vi "串口发送.vi"(6 "写入缓冲区":string, 7 "命令":string(combo), 8 "error in (no error)":errorcluster caption="错误输入（无错误）", 10 "baud rate (9600)":u32=115200 caption="波特率(115200)", 11 "VISA resource name":refnum<visa-resource-name> caption="VISA资源名称") -> (0 "错误输出":errorcluster, 3 "VISA resource name 2":refnum<visa-resource-name>, 4 "读取缓冲区":string)   [LabVIEW 2016]
uses:
  <vilib>/Instr/_visa.llb/VISA Flush IO Buffer Mask.ctl
  <vilib>/Instr/_visa.llb/VISA Configure Serial Port (Instr).vi
panel:
  in  "timeout (10sec)":u32=10000 caption="超时（10秒）"
  out "返回数":u32
  in  "parity (0:none)":enum16{"None", "Odd", "Even", "Mark", "Space"}(ring) caption="奇偶（0:无）"
  in  "data bits (8)":u16=8 caption="数据比特(8)" min=5 max=8 step=1
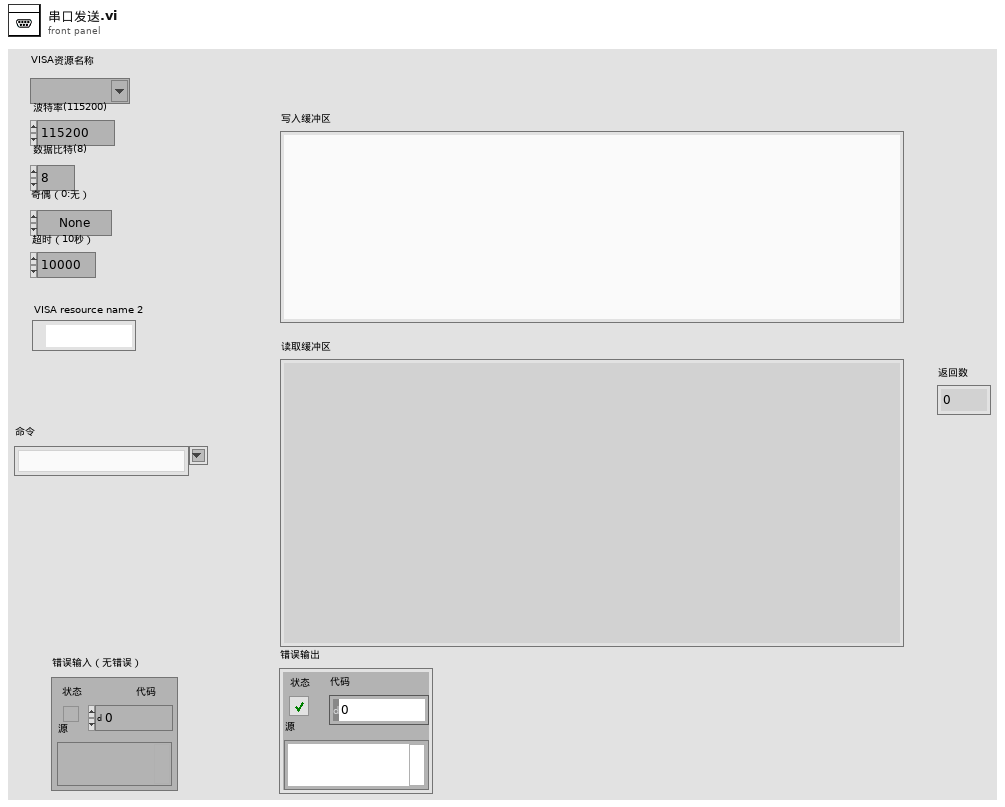
[diagram p1: front panel]
types:
  T1 = typedef "VISA Flush IO Buffer Mask.ctl" = u16
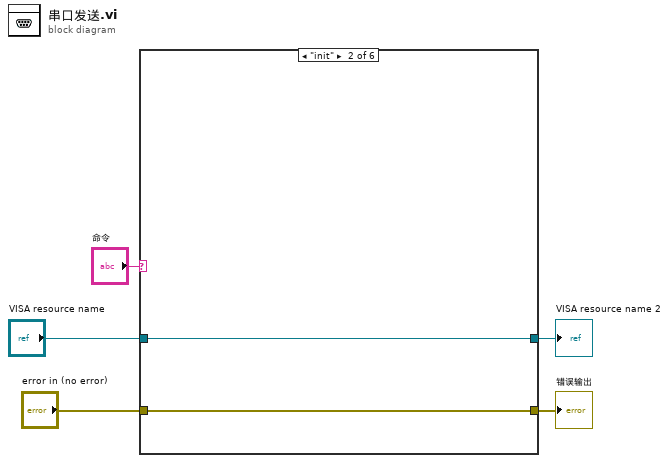
[diagram p0: block diagram]
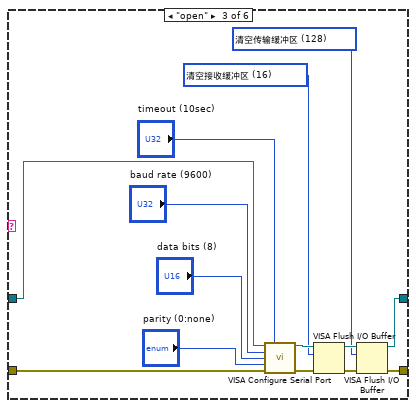
[diagram p3: hidden frame]
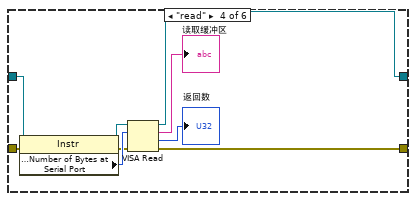
[diagram p4: hidden frame]
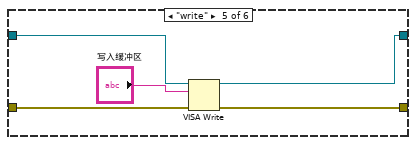
[diagram p5: hidden frame]
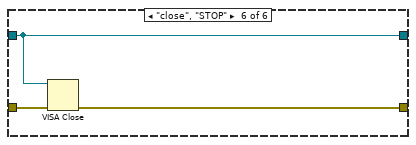
[diagram p6: hidden frame]
diagram:
  n1 = case shown="\"init\"" "命令" {
    tunnel: "error in (no error)" -> [w7 w9 w20 w31 w36 w40]
    tunnel: [w7 w9 w12 w25 w35 w39] -> w3
    tunnel: "VISA resource name" -> [w6 w8 w11 w32 w37 w38]
    tunnel: [w6 w8 w10 w24 w33 w38] -> w1
    frame "idle", Default {
    }
    frame "init" {
    }
    frame "open" {
      w13 = T1 128 items=["清空接收缓冲区"=16, "向设备写入传输缓冲区"=32, "清空接收缓冲区（无I/O）"=64, "清空传输缓冲区"=128] ("Mask")
      w16 = T1 16 items=["清空接收缓冲区"=16, "向设备写入传输缓冲区"=32, "清空接收缓冲区（无I/O）"=64, "清空传输缓冲区"=128] ("Mask")
      n2 = call-poly "VISA Configure Serial Port"("VISA resource name"=w11, "timeout (10sec)"="timeout (10sec)", "baud rate (9600)"="baud rate (9600)", "data bits (8)"="data bits (8)", "parity (0:none)"="parity (0:none)", "error in (no error)"=w20) -> ("VISA resource name out"=w18:refnum<visa-resource-name>, "error out"=w19:errorcluster)  [unwired: 8 in]
      n3 = VISA Flush I/O Buffer(VISA resource name=w18, mask (16)=w16, error in (no error)=w19) -> (VISA resource name out=w14:refnum<visa-resource-name>, error out=w15:errorcluster)
      n4 = VISA Flush I/O Buffer(VISA resource name=w14, mask (16)=w13, error in (no error)=w15) -> (VISA resource name out=w10:refnum<visa-resource-name>, error out=w12:errorcluster)
    }
    frame "read" {
      n5 = property class="Instr"(reference=w32, error in=w31) -> (reference out=w28:refnum<visa-resource-name>, error out=w29:errorcluster, "Serial Settings:Number of Bytes at Serial Port"=w30:u32)
      n6 = VISA Read(VISA resource name=w28, byte count=w30, error in (no error)=w29) -> (VISA resource name out=w24:refnum<visa-resource-name>, read buffer=→"读取缓冲区":string, return count=→"返回数":u32, error out=w25:errorcluster)
    }
    frame "write" {
      n7 = VISA Write(VISA resource name=w37, write buffer="写入缓冲区", error in (no error)=w36) -> (VISA resource name out=w33:refnum<visa-resource-name>, error out=w35:errorcluster)  [unwired: 1 out]
    }
    frame "close", "STOP" {
      n8 = VISA Close(VISA resource name=w38, error in (no error)=w40) -> (error out=w39:errorcluster)
    }
  }
  "错误输出" <- w3
  "VISA resource name 2" <- w1
